vi "Read Channel Info No Objects.vi"(8 "error in (no error)":errorcluster, 11 "Synapse CCD in":T1={"JYCCDLib.IJYCCDReqd"=refnum, "JYMONOLib.IJYMonoReqd"=refnum, "Integration time"=0.01, "ADC"=0, "GAIN"=0, "areas :"=[[1, 1, 1, 1024, 256, 1, 256]], "Most Recent Data Object"=refnum, "Mono Properties"={"Grating"=0, "Center Wavelength"=0.0, "Entrance Slit"=0.0, "Exit Slit"=0.0}, "Coverage"={"Max"=0.0, "Min"=0.0}, "Multi-Acquisitions"={"Dark Subtract?"=FALSE, "Averaging?"=FALSE, "Cosmic Ray Removal?"=FALSE, "# to Average"=0, "Time Between Acq."=0, "Acquisitions Control Array"=[TRUE], "Raw Data"=[], "Processed Data"=[], "Array of Wavelengths"=[]}, "Channel Names"=["Wavelength", "Signal"], "Channel Units"=["nm", "counts"]} {"ADC" items=["   20 kHz", "1 MHz", "1 MHz Ultra"]; "GAIN" items=["High Light", "Best Dynamic", "High Sensitivity"]; "Mono Properties"."Grating" items=["1200 lines/mm - 500 nm Blaze", "1200 lines/mm - 750 nm Blaze", "600 lines/mm - 1000 nm Blaze"]}) -> (0 "error out":errorcluster, 1 "Channel Units":string[](array[string]), 2 "Channel Names":string[](array[string]), 3 "Synapse CCD out":T1={"JYCCDLib.IJYCCDReqd"=refnum, "JYMONOLib.IJYMonoReqd"=refnum, "Integration time"=0.01, "ADC"=0, "GAIN"=0, "areas :"=[[1, 1, 1, 1024, 256, 1, 256]], "Most Recent Data Object"=refnum, "Mono Properties"={"Grating"=0, "Center Wavelength"=0.0, "Entrance Slit"=0.0, "Exit Slit"=0.0}, "Coverage"={"Max"=0.0, "Min"=0.0}, "Multi-Acquisitions"={"Dark Subtract?"=FALSE, "Averaging?"=FALSE, "Cosmic Ray Removal?"=FALSE, "# to Average"=0, "Time Between Acq."=0, "Acquisitions Control Array"=[TRUE], "Raw Data"=[], "Processed Data"=[], "Array of Wavelengths"=[]}, "Channel Names"=["Wavelength", "Signal"], "Channel Units"=["nm", "counts"]} {"ADC" items=["   20 kHz", "1 MHz", "1 MHz Ultra"]; "GAIN" items=["High Light", "Best Dynamic", "High Sensitivity"]; "Mono Properties"."Grating" items=["1200 lines/mm - 500 nm Blaze", "1200 lines/mm - 750 nm Blaze", "600 lines/mm - 1000 nm Blaze"]}, 5 "#Channels":i32)   [LabVIEW 2015]
doc: "(Dynamic) Return information about the readable data channels this object provides, e.g., the name of each data source and its unit."
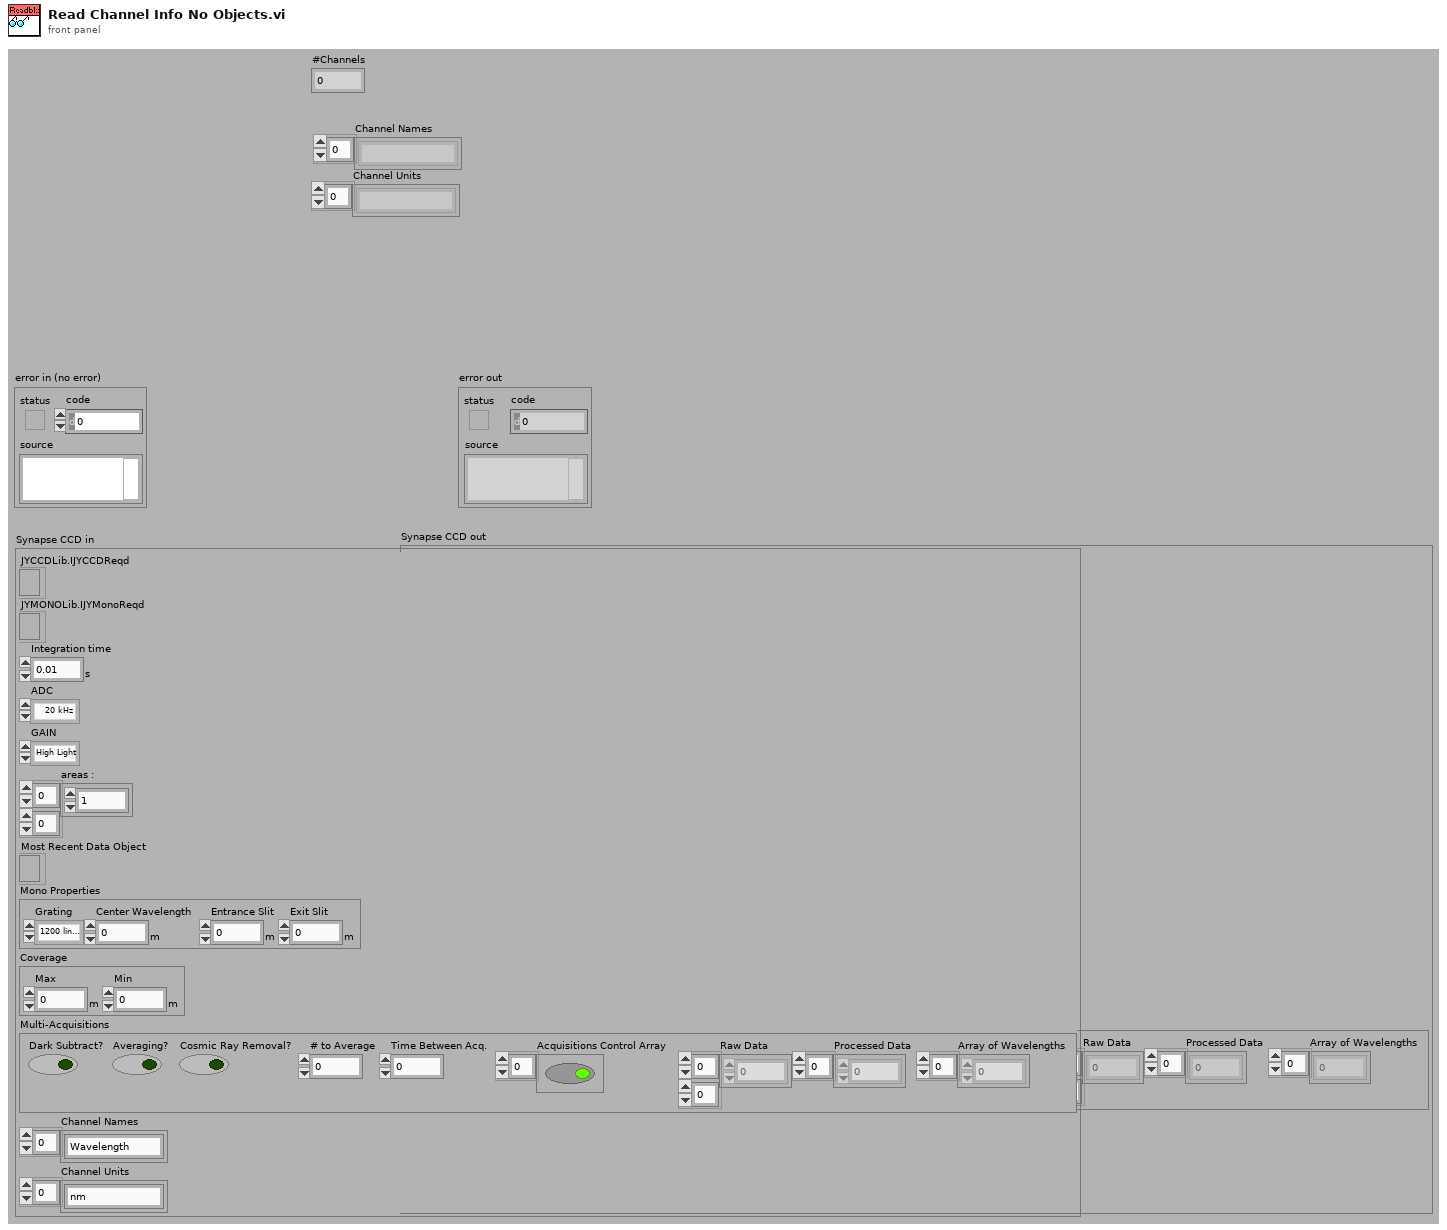
[diagram p1: front panel]
types:
  T1 = cluster{"JYCCDLib.IJYCCDReqd":refnum<k7>, "JYMONOLib.IJYMonoReqd":refnum<k7>, "Integration time":dbl[unit], "ADC":u16, "GAIN":u16, "areas :":i32[][], "Most Recent Data Object":refnum<k7>, "Mono Properties":cluster{"Grating":u16, "Center Wavelength":dbl[unit], "Entrance Slit":dbl[unit], "Exit Slit":dbl[unit]}, "Coverage":cluster{"Max":dbl[unit], "Min":dbl[unit]}, "Multi-Acquisitions":cluster{"Dark Subtract?":bool, "Averaging?":bool, "Cosmic Ray Removal?":bool, "# to Average":u32, "Time Between Acq.":u32, "Acquisitions Control Array":bool[], "Raw Data":i32[][], "Processed Data":dbl[], "Array of Wavelengths":dbl[]}, "Channel Names":string[], "Channel Units":string[]}
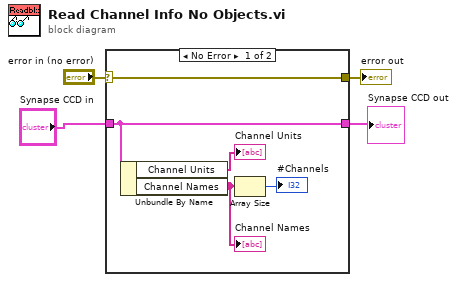
[diagram p0: block diagram]
diagram:
  n1 = case shown="No Error" "error in (no error)" {
    selector: "error in (no error)" -> [w8 w10]
    tunnel: [w8 w10] -> w3
    tunnel: [w6 w11] -> w2
    tunnel: "Synapse CCD in" -> [w6 w11]
    frame No Error {
      n2 = Unbundle By Name(w6) -> ("Channel Units"=→"Channel Units":string[], "Channel Names"=w5:string[])
      "Channel Names" <- w5
      n3 = Array Size(array=w5) -> (size(s)=→"#Channels":i32)
    }
    frame Error {
    }
  }
  "error out" <- w3
  "Synapse CCD out" <- w2
